vi "SignalGenerator.vi"(1 "stop":bool, 2 "Amplitude":i32=2, 3 "Frequency":i32=10) -> ()   [LabVIEW 2015]
panel:
  out "error in":errorcluster
  out "error out":errorcluster
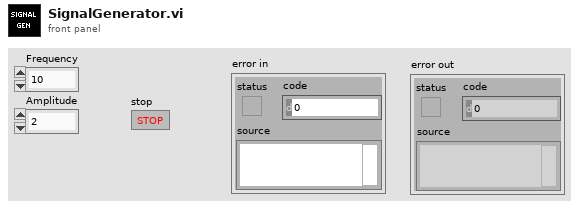
[diagram p1: front panel]
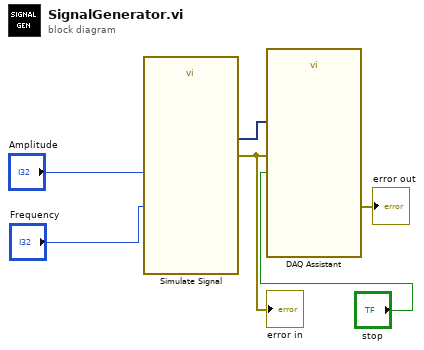
[diagram p0: block diagram]
diagram:
  n1 = call "Simulate Signal"("Frequency"="Frequency", "Amplitude"="Amplitude") -> ("Sine"=w4:dynamicdata, "error out"=w2:errorcluster)  [unwired: 12 in]
  "error in" <- w2
  n2 = call "DAQ Assistant"("data"=w4, "error in"=w2, "stop (F)"="stop") -> ("error out"=→"error out":errorcluster)  [unwired: 14 in, 2 out]
